vi "testing mc listbox customization.vi"() -> ()   [LabVIEW 2021]
uses:
  <vilib>/Utility/miscctls.llb/LVRowAndColumnUnsignedTypeDef.ctl
  <vilib>/Utility/miscctls.llb/LVRowAndColumnTypeDef.ctl
panel:
  out "size(s)":i32[](array[numeric])
  out "error out":errorcluster
  out "x-y*floor(x/y)":i32
  in  "Stop":bool
  in  "Multicolumn Listbox":i32(listbox)
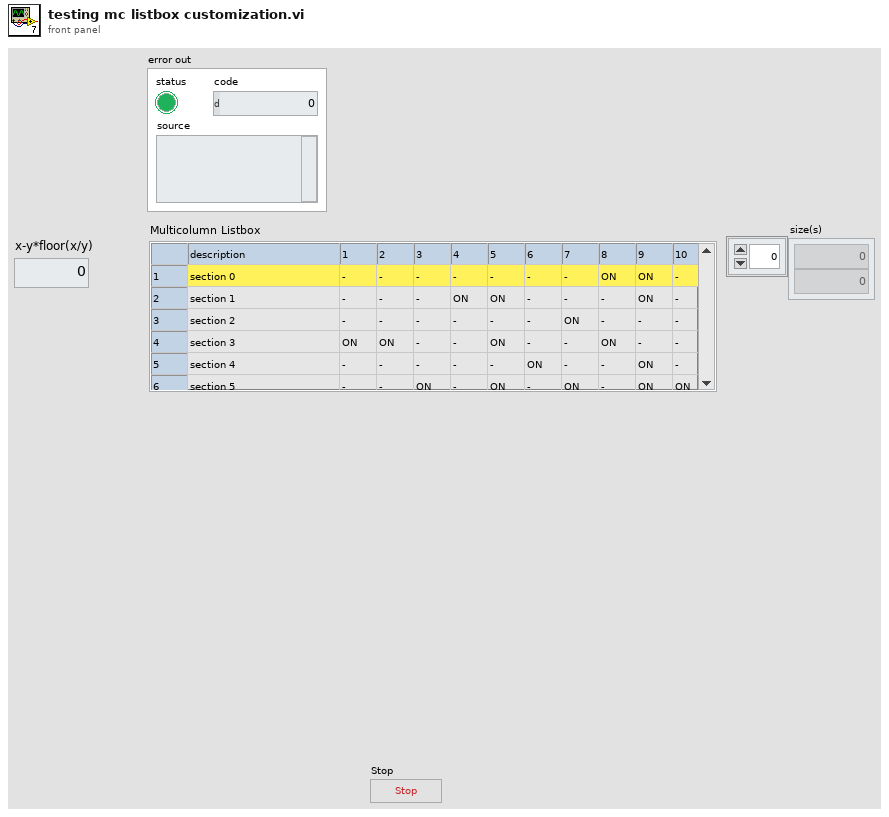
[diagram p1: front panel]
types:
  T1 = typedef "LVRowAndColumnTypeDef.ctl" = cluster{"Row":i32, "Column":i32}
  T2 = typedef "LVRowAndColumnUnsignedTypeDef.ctl" = cluster{"Row":u32, "Column":u32}
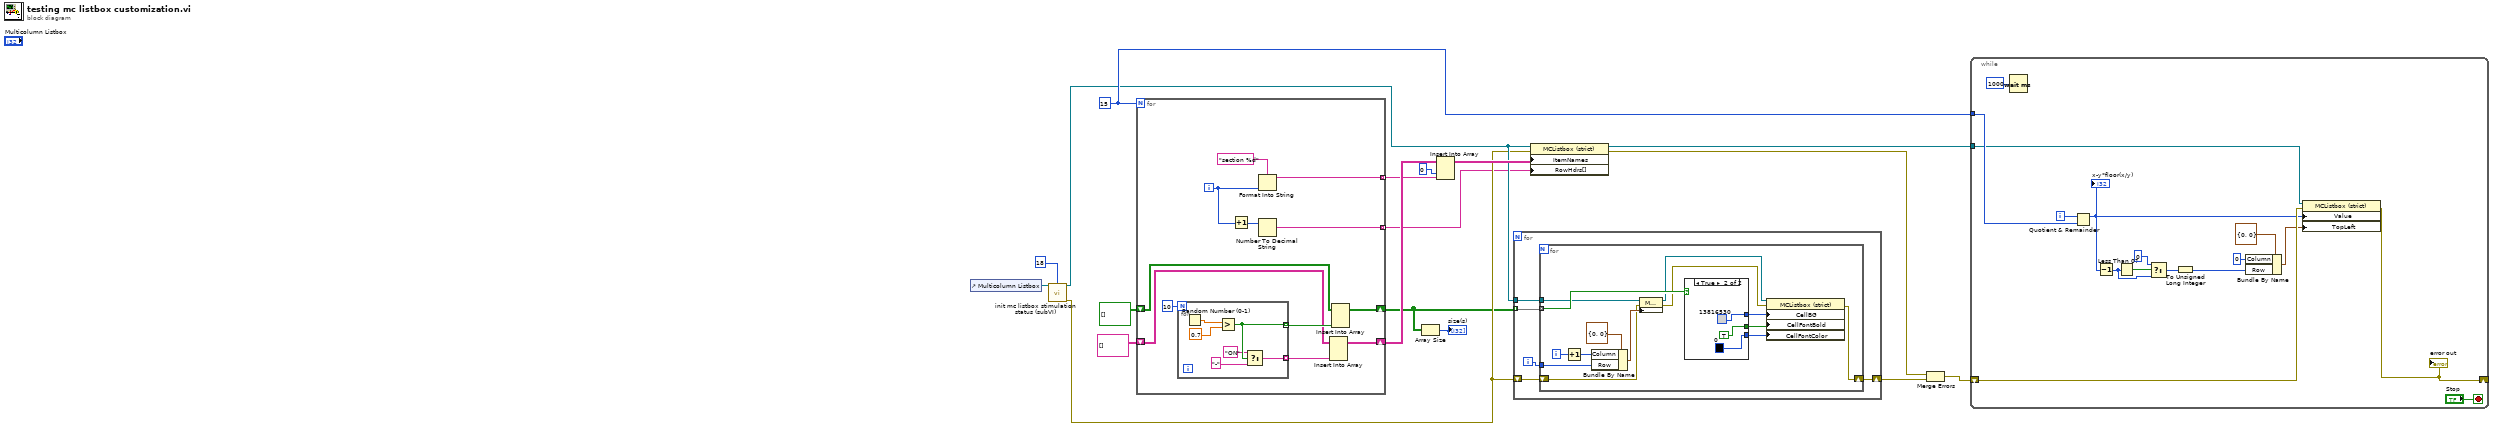
[diagram p0: block diagram]
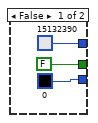
[diagram p2: hidden frame]
diagram:
  w17 = 15
  n1 = control-ref of="Multicolumn Listbox"() -> (w18:refnum<vi>)
  n2 = call "init mc listbox stimulation status (subVI).vi"("mc listbox refnum"=w18, "font size (16)"=u32 18) -> ("mc listbox refnum out"=w6:refnum<vi>, "error out"=w5:errorcluster)  [unwired: 12 in]
  n3 = for {
    N: w17 -> [_]
    tunnel: [w29] -> w9 mode=indexing
    shift-right: [w28] -> w3
    shift-left: bool[][] [] -> [w24]
    shift-right: [w25] -> w10
    shift-left: string[][] [] -> [w23]
    tunnel: [w21] -> w4 mode=indexing
    i -> [w22]
    n4 = for {
      N: 10 -> [_]
      tunnel: [w34] -> w27 mode=indexing
      tunnel: [w31] -> w26 mode=indexing
      n5 = Random Number (0-1)() -> (number: 0 to 1=w36:dbl)
      n6 = Greater?(x=w36, y=0.7) -> (0:w34:bool)
      n7 = Select(t="ON", s=w34, f="-") -> (s? t:f=w31:string)
    }
    n8 = Increment(x=w22) -> (x+1=w20:i32)
    n9 = Format Into String(format string="section %d", w22) -> (resulting string=w29:string)  [unwired: 2 in, 1 out]
    n10 = Number To Decimal String(number=w20) -> (decimal integer string=w21:string)  [unwired: 1 in]
    n11 = Insert Into Array(array=w23, new element=w26) -> (w25:string[][])  [unwired: 2 in]
    n12 = Insert Into Array(array=w24, new element=w27) -> (w28:bool[][])  [unwired: 2 in]
  }
  n13 = Array Size(array=w3) -> (size(s)=→"size(s)":i32[])
  n14 = Insert Into Array(array=w10, index (col)=0 ("disabled index (col)"), new element=w9) -> (w8:string[][])  [unwired: 1 in]
  n15 = for {
    tunnel: w3 -> [w41] mode=indexing
    shift-right: [w39] -> w14
    shift-left: w5 -> [w38]
    tunnel: w6 -> [w37]
    i -> [w40]
    n16 = for {
      tunnel: w41 -> [w51] mode=indexing
      tunnel: w40 -> [w54]
      shift-right: [w44] -> w39
      shift-left: w38 -> [w45]
      tunnel: w37 -> [w43]
      i -> [w55]
      n17 = Increment(x=w55) -> (x+1=w42:i32)
      n18 = Bundle By Name(cluster=T1 {"Row"=0, "Column"=0} ("Active Cell:Active Cell"), "Column"=w42, "Row"=w54) -> (w52:T1)
      n19 = property on="Property Node" class="MCListbox (strict)"(reference=w43, error in=w45, "ActiveCell"=w52) -> (reference out=w47:refnum<vi>, error out=w46:errorcluster)
      n20 = case shown="True" w51 {
        tunnel: [FALSE ("Active Cell:Cell Font:Bold") TRUE ("Active Cell:Cell Font:Bold")] -> w50
        tunnel: [u32 15132390 ("Selection Color") u32 13816530 ("Selection Color")] -> w49
        tunnel: [u32 0 ("Selection Color") u32 0 ("Selection Color")] -> w48
        frame False {
        }
        frame True {
        }
      }
      n21 = property on="Property Node" class="MCListbox (strict)"(reference=w47, error in=w46, "CellBG"=w49, "CellFontBold"=w50, "CellFontColor"=w48) -> (error out=w44:errorcluster)  [unwired: 1 out]
    }
  }
  n22 = property on="Property Node" class="MCListbox (strict)"(reference=w6, error in=w5, "ItemNames"=w8, "RowHdrs[]"=w4) -> (reference out=w11:refnum<vi>, error out=w13:errorcluster)
  n23 = Merge Errors(w13, w14) -> (w12:errorcluster)
  n24 = while {
    shift-right: [w73] -> _
    shift-left: w12 -> [w74]
    tunnel: w17 -> [w72]
    tunnel: w11 -> [w71]
    i -> [w76]
    stop <- "Stop" stop-if-true
    n25 = Wait (ms)(milliseconds to wait=u32 1000) -> ()  [unwired: 1 out]
    n26 = Quotient & Remainder(x=w76, y=w72) -> (x-y*floor(x/y)=w69:i32)  [unwired: 1 out]
    "x-y*floor(x/y)" <- w69
    n27 = Decrement(x=w69) -> (x-1=w65:i32)
    n28 = Less Than 0?(x=w65) -> (x < 0?=w66:bool)
    n29 = Select(t=0, s=w66, f=w65) -> (s? t:f=w63:i32)
    n30 = To Unsigned Long Integer(number=w63) -> (unsigned 32bit integer=w62:u32)
    n31 = Bundle By Name(cluster=T2 {"Row"=0, "Column"=0} ("Top Left Visible Cell"), "Column"=u32 0, "Row"=w62) -> (w67:T2)
    n32 = property on="Property Node" class="MCListbox (strict)"(reference=w71, error in=w74, "Value"=w69, "TopLeft"=w67) -> (error out=w73:errorcluster)  [unwired: 1 out]
    "error out" <- w73
  }
